vi "InvalidConfig.vi"() -> (1 "status":string="ok")   [LabVIEW 2017, in "ChannelStatus.lvlib"]
uses:
  <vilib>/addons/InsightCM/Utilities/ChannelStatus/ChannelStatus.lvlib
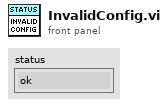
[diagram p1: front panel]
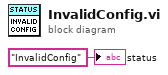
[diagram p0: block diagram]
diagram:
  "status" <- "InvalidConfig"
